vi "Read-Network.vi"(8 "error in (no error)":errorcluster, 11 "Refnum in":T2) -> (0 "error out":errorcluster, 2 "Network":T1, 3 "Refnum out":T2)   [LabVIEW 2021, in "UDP_Config.lvclass"]
uses:
  UDP_Config.lvclass
  <vilib>/Utility/config.llb/Config Data RefNum.ctl
  Network.ctl
  <vilib>/Utility/config.llb/Read Key (String).vi
  <vilib>/Utility/config.llb/Read Key (I32).vi
  <vilib>/Utility/config.llb/NI_LVConfig.lvlib
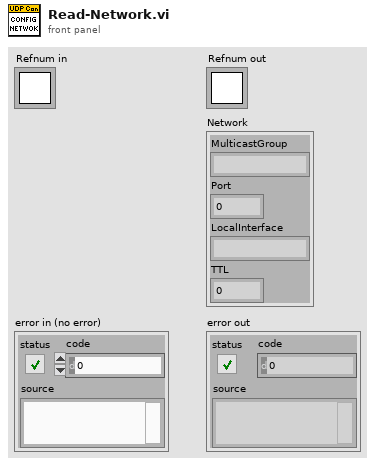
[diagram p1: front panel]
types:
  T1 = typedef "Network.ctl" = cluster{"MulticastGroup":string, "Port":u16, "LocalInterface":string, "TTL":u8}
  T2 = typedef "NI_LVConfig.lvlib/Config Data RefNum.ctl" = refnum<k1>
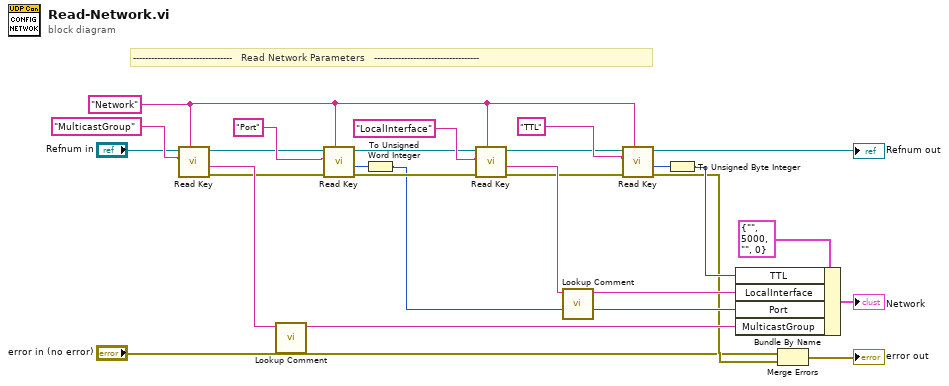
[diagram p0: block diagram]
diagram:
  w21 = "Network" ("key")
  # "---------------------------------   Read Network Parameters   -----------------------------------"
  n1 = call-poly <vilib>:"Read Key.vi"("section"=w21, "key"="MulticastGroup", "refnum"="Refnum in") -> ("error out"=w13:errorcluster, "value"=w25:string, "refnum out"=w12:T2)  [unwired: 5 in, 1 out]
  n2 = call "Lookup Comment.vi"("String in"=w25) -> ("Value"=w7:string)  [unwired: 3 in, 1 out]
  n3 = call-poly <vilib>:"Read Key.vi"("section"=w21, "error in (no error)"=w13, "key"="Port", "refnum"=w12) -> ("error out"=w17:errorcluster, "value"=w15:i32, "refnum out"=w16:T2)  [unwired: 4 in, 1 out]
  n4 = To Unsigned Word Integer(number=w15) -> (unsigned 16bit integer=w6:u16)
  n5 = call-poly <vilib>:"Read Key.vi"("section"=w21, "error in (no error)"=w17, "key"="LocalInterface", "refnum"=w16) -> ("error out"=w19:errorcluster, "value"=w26:string, "refnum out"=w20:T2)  [unwired: 4 in, 1 out]
  n6 = call "Lookup Comment.vi"("String in"=w26) -> ("Value"=w5:string)  [unwired: 3 in, 1 out]
  n7 = call-poly <vilib>:"Read Key.vi"("section"=w21, "error in (no error)"=w19, "key"="TTL", "refnum"=w20) -> ("error out"=w2:errorcluster, "value"=w22:i32, "refnum out"=→"Refnum out":T2)  [unwired: 4 in, 1 out]
  n8 = To Unsigned Byte Integer(number=w22) -> (unsigned 8bit integer=w4:u8)
  n9 = Bundle By Name(cluster=T1 {"MulticastGroup"="", "Port"=5000, "LocalInterface"="", "TTL"=0} ("Network"), "TTL"=w4, "LocalInterface"=w5, "Port"=w6, "MulticastGroup"=w7) -> (→"Network":T1)
  n10 = Merge Errors("error in (no error)", w2) -> (→"error out":errorcluster)
